vi "Stop Test to Plugins.vi"(8 "error in (no error)":errorcluster, 11 "Execution API in":refnum<class "Execution API.lvclass">) -> (0 "error out":errorcluster, 3 "Execution API out":refnum<class "Execution API.lvclass">)   [LabVIEW 2020]
uses:
  Framework/Plugin/Plugin.lvclass
  Execution API.lvclass
  C:/git/astemes-lunit/source/User Interface/Execution API/Execution API.lvclass
  C:/git/astemes-lunit/source/Framework/Result Observer/Result Observer.lvclass
  C:/git/astemes-lunit/source/Framework/Plugin/Plugin.lvclass
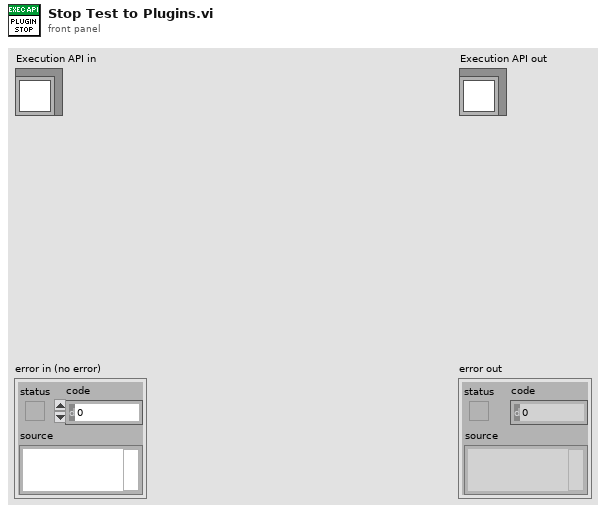
[diagram p1: front panel]
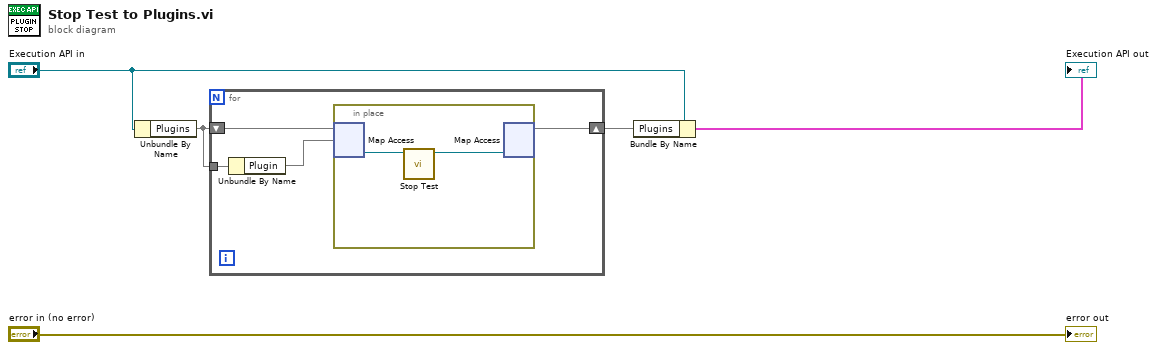
[diagram p0: block diagram]
diagram:
  n1 = Unbundle By Name("Execution API in") -> ("Plugins"=w3)
  n2 = for {
    shift-right: [w6] -> w1
    shift-left: w3 -> [w9]
    tunnel: w3 -> [w8]
    n3 = Unbundle By Name(w8) -> ("Plugin"=w7)
    n4 = in-place {
      n5 = in-place-map #1(w9, w7) -> (w11:refnum<class "Plugin.lvclass">)  [unwired: 1 in, 1 out]
      n6 = call-dynamic "Stop Test.vi"("Plugin in"=w11) -> ("Plugin out"=w10:refnum<class "Plugin.lvclass">)  [unwired: 9 in, 1 out]
      n7 = in-place-map #1(w10) -> (w6:map{string, refnum<class "Plugin.lvclass">})  [unwired: 1 in, 2 out]
    }
  }
  n8 = Bundle By Name(cluster="Execution API in", "Plugins"=w1) -> (→"Execution API out":cluster{})
  "error out" <- "error in (no error)"
